vi "niRFUtil ERR Check Valid Input Exclude Limits (DBL).vi"(0 "Property Value":dbl format="%_3p", 1 "Property Name":string, 7 "Upper Limit":dbl=inf, 9 "Lower Limit":dbl=-inf, 11 "error in (no error)":errorcluster, 12 "Error Code":i32=-379001) -> (15 "error out":errorcluster)   [LabVIEW 2015, in "niRFUtil.lvlib"]
uses:
  niRFUtil.lvlib
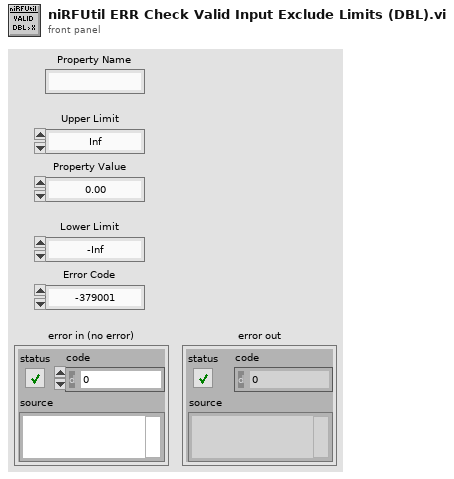
[diagram p1: front panel]
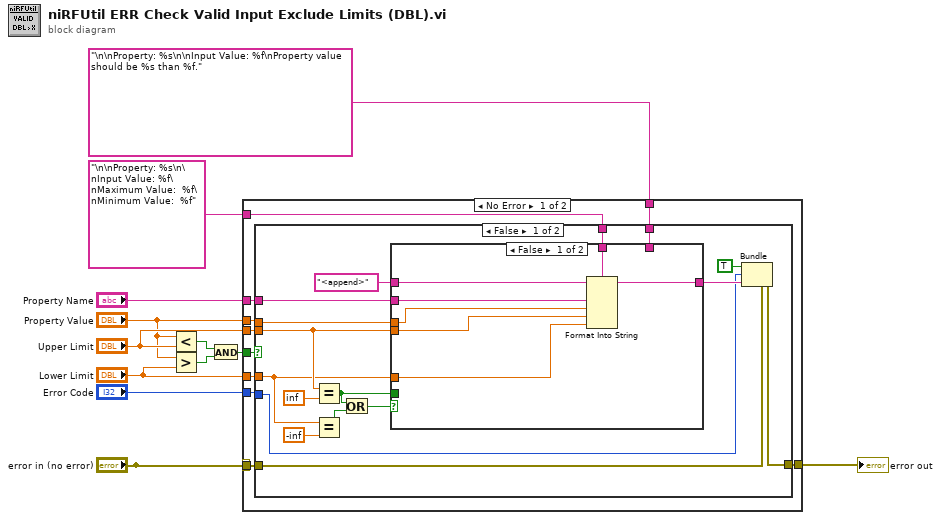
[diagram p0: block diagram]
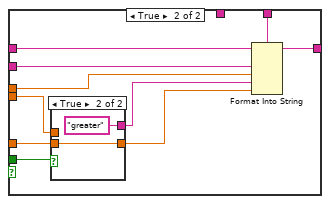
[diagram p2: hidden frame]
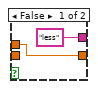
[diagram p3: hidden frame]
diagram:
  n1 = Less?(x="Property Value", y="Upper Limit") -> (x < y?=w4:bool)
  n2 = Greater?(x="Property Value", y="Lower Limit") -> (0:w3:bool)
  n3 = And(x=w4, y=w3) -> (x .and. y?=w2:bool)
  n4 = case shown="No Error" "error in (no error)" {
    tunnel: "\n\nProperty: %s\n\nInput Value: %f\nMaximum Value:  %f\nMinimum Value:  %f" ("initial string") -> [w22 _]
    tunnel: "\n\nProperty: %s\n\nInput Value: %f\nProperty value should be %s than %f." ("initial string") -> [w21 _]
    tunnel: "Property Name" -> [w20 _]
    tunnel: "Error Code" -> [w19 _]
    tunnel: "error in (no error)" -> [w18 w62]
    tunnel: [w17 w62] -> w8
    tunnel: "Lower Limit" -> [w16 _]
    tunnel: "Upper Limit" -> [w15 _]
    tunnel: "Property Value" -> [w14 _]
    tunnel: w2 -> [w13 _]
    frame No Error {
      n5 = case shown="False" w13 {
        tunnel: w22 -> [w36 _]
        tunnel: w14 -> [w39 _]
        tunnel: w15 -> [w32 _]
        tunnel: w16 -> [w31 _]
        tunnel: w20 -> [w38 _]
        tunnel: w19 -> [w24 _]
        tunnel: w18 -> [w26 w61]
        tunnel: [w37 w61] -> w17
        tunnel: w21 -> [w35 _]
        frame False {
          n6 = Equal?(x=w32, y=inf) -> (x = y?=w28:bool)
          n7 = Equal?(x=w31, y=-inf) -> (x = y?=w29:bool)
          n8 = Or(x=w28, y=w29) -> (x .or. y?=w30:bool)
          n9 = case shown="False" w30 {
            tunnel: w39 -> [w46 w52]
            tunnel: w32 -> [w45 w49]
            tunnel: w31 -> [w44 w50]
            tunnel: w38 -> [w43 w53]
            tunnel: "<append>" ("message") -> [w42 w56]
            tunnel: [w40 w54] -> w25
            tunnel: w36 -> [w41 _]
            tunnel: w35 -> [_ w55]
            tunnel: w28 -> [_ w47]
            frame False {
              n10 = Format Into String(format string=w41, initial string=w42, w43, w46, w45, w44) -> (resulting string=w40:string)  [unwired: 1 in, 1 out]
            }
            frame True {
              n11 = case shown="True" w47 {
                tunnel: ["less" ("initial string") "greater" ("initial string")] -> w51
                tunnel: w50 -> [_ w59]
                tunnel: w49 -> [w57 _]
                tunnel: [w57 w59] -> w48
                frame False {
                }
                frame True {
                }
              }
              n12 = Format Into String(format string=w55, initial string=w56, w53, w52, w51, w48) -> (resulting string=w54:string)  [unwired: 1 in, 1 out]
            }
          }
          n13 = Bundle(cluster=w26, "status"=TRUE, "code"=w24, "source"=w25) -> (w37:errorcluster)
        }
        frame True {
        }
      }
    }
    frame Error {
    }
  }
  "error out" <- w8
